vi "SP Get Cluster Element Reference.vi"(4 "Channel":i8=1 min=1 max=99 step=1, 5 "Element":T1, 7 "Plot Reference":refnum<vi>) -> (1 "Element Reference":refnum<vi>)   [LabVIEW 2011]
uses:
  TypeDefs/SP Plot Cluster Object.ctl
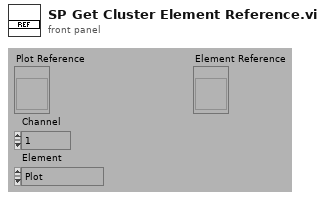
[diagram p1: front panel]
types:
  T1 = typedef "SP Plot Cluster Object.ctl" = enum16{"Plot", "CH Reference", "CH Label", "Start Label", "Stop Label", "Units Label", "Selected?", "CH Markers"}
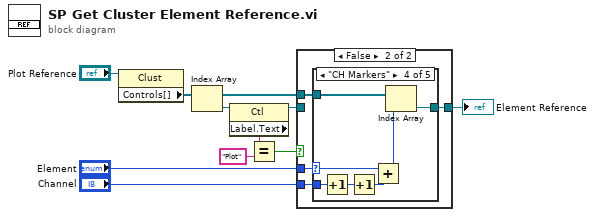
[diagram p0: block diagram]
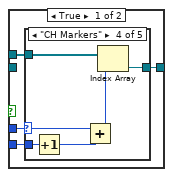
[diagram p2: hidden frame]
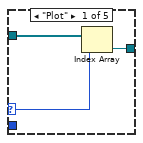
[diagram p3: hidden frame]
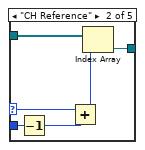
[diagram p4: hidden frame]
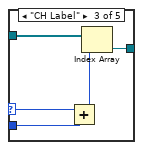
[diagram p5: hidden frame]
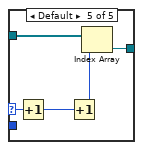
[diagram p6: hidden frame]
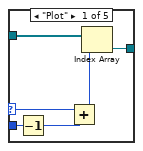
[diagram p7: hidden frame]
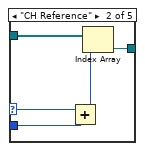
[diagram p8: hidden frame]
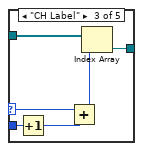
[diagram p9: hidden frame]
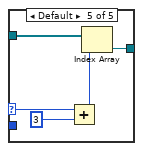
[diagram p10: hidden frame]
diagram:
  n1 = property class="Clust"(reference="Plot Reference") -> ("Controls[]"=w3:refnum<vi>[])  [unwired: 1 in, 2 out]
  n2 = Index Array(array=w3) -> (element=w8:refnum<vi>)  [unwired: 1 in]
  n3 = property class="Ctl"(reference=w8) -> (reference out=w4:refnum<vi>, "Label.Text"=w7:string)  [unwired: 1 in, 1 out]
  n4 = Equal?(x=w7, y="Plot") -> (x = y?=w5:bool)
  n5 = case shown="False" w5 {
    tunnel: w4 -> [_ _]
    tunnel: [w13 w42] -> w9
    tunnel: w3 -> [w14 w41]
    tunnel: "Element" -> [w11 w43]
    tunnel: "Channel" -> [w12 w40]
    frame True {
      n6 = case shown="\"CH Markers\"" w11 {
        selector: w11 -> [w15 w20 w26 w31 w35]
        tunnel: w14 -> [w17 w23 w28 w34 w39]
        tunnel: [w16 w22 w27 w33 w38] -> w13
        tunnel: w12 -> [_ w21 w24 w32 _]
        frame "Plot" {
          n7 = Index Array(array=w17, index=w15) -> (element=w16:refnum<vi>)
        }
        frame "CH Reference" {
          n8 = Decrement(x=w21) -> (x-1=w19:i8)
          n9 = Add(x=w20, y=w19) -> (x+y=w18:u16)
          n10 = Index Array(array=w23, index=w18) -> (element=w22:refnum<vi>)
        }
        frame "CH Label" {
          n11 = Add(x=w26, y=w24) -> (x+y=w25:u16)
          n12 = Index Array(array=w28, index=w25) -> (element=w27:refnum<vi>)
        }
        frame "CH Markers" {
          n13 = Increment(x=w32) -> (x+1=w30:i8)
          n14 = Add(x=w31, y=w30) -> (x+y=w29:u16)
          n15 = Index Array(array=w34, index=w29) -> (element=w33:refnum<vi>)
        }
        frame Default {
          n16 = Increment(x=w35) -> (x+1=w36:T1)
          n17 = Increment(x=w36) -> (x+1=w37:T1)
          n18 = Index Array(array=w39, index=w37) -> (element=w38:refnum<vi>)
        }
      }
    }
    frame False {
      n19 = case shown="\"CH Markers\"" w43 {
        selector: w43 -> [w46 w52 w58 w65 w69]
        tunnel: w41 -> [w49 w54 w60 w67 w72]
        tunnel: [w48 w53 w59 w66 w71] -> w42
        tunnel: w40 -> [w47 w50 w56 w63 _]
        frame "Plot" {
          n20 = Decrement(x=w47) -> (x-1=w45:i8)
          n21 = Add(x=w46, y=w45) -> (x+y=w44:u16)
          n22 = Index Array(array=w49, index=w44) -> (element=w48:refnum<vi>)
        }
        frame "CH Reference" {
          n23 = Add(x=w52, y=w50) -> (x+y=w51:u16)
          n24 = Index Array(array=w54, index=w51) -> (element=w53:refnum<vi>)
        }
        frame "CH Label" {
          n25 = Increment(x=w56) -> (x+1=w55:i8)
          n26 = Add(x=w58, y=w55) -> (x+y=w57:u16)
          n27 = Index Array(array=w60, index=w57) -> (element=w59:refnum<vi>)
        }
        frame "CH Markers" {
          n28 = Increment(x=w63) -> (x+1=w62:i8)
          n29 = Increment(x=w62) -> (x+1=w61:i8)
          n30 = Add(x=w65, y=w61) -> (x+y=w64:u16)
          n31 = Index Array(array=w67, index=w64) -> (element=w66:refnum<vi>)
        }
        frame Default {
          n32 = Add(x=w69, y=3) -> (x+y=w70:i32)
          n33 = Index Array(array=w72, index=w70) -> (element=w71:refnum<vi>)
        }
      }
    }
  }
  "Element Reference" <- w9
